vi "FindKeywords.vi"(9 "After":string, 11 "Before":string) -> (2 "Cmd?":bool)   [LabVIEW 2020]
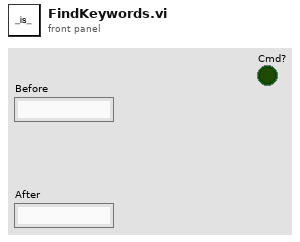
[diagram p1: front panel]
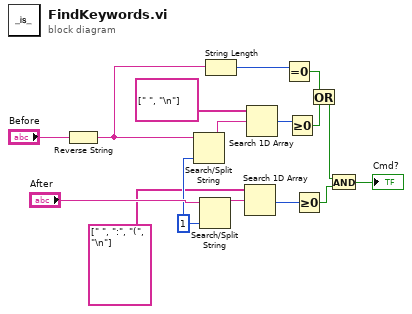
[diagram p0: block diagram]
diagram:
  w11 = 1 ("offset (0)")
  n1 = Reverse String(1:"Before") -> (0:w7:string)
  n2 = Search/Split String(string=w7, offset (0)=w11) -> (substring before match=w9:string)  [unwired: 1 in, 2 out]
  n3 = Search/Split String(string="After", offset (0)=w11) -> (substring before match=w15:string)  [unwired: 1 in, 2 out]
  n4 = String Length(string=w7) -> (length=w6:i32)
  n5 = Search 1D Array(1D array=string[] [" ", ":", "(", "\n"], element=w15) -> (index of element=w13:i32)  [unwired: 1 in]
  n6 = Search 1D Array(1D array=string[] [" ", "\n"], element=w9) -> (index of element=w8:i32)  [unwired: 1 in]
  n7 = Equal To 0?(x=w6) -> (x = 0?=w5:bool)
  n8 = Greater Or Equal To 0?(x=w8) -> (x >= 0?=w4:bool)
  n9 = Greater Or Equal To 0?(x=w13) -> (x >= 0?=w12:bool)
  n10 = Or(x=w5, y=w4) -> (x .or. y?=w3:bool)
  n11 = And(x=w3, y=w12) -> (x .and. y?=→"Cmd?":bool)
